vi "DriverStationPushData.vi"   [LabVIEW 2020]
doc: "This VI continously sends data from the robot to the FRC 4265 Dashboard, the joysticks, and the FIRST Driver Station. Data are only sent to the network tables when values change. Detailed sensor data are only sent when the user is currently viewing the Tune tab on the FRC 4265 Dashboard."
uses:
  04c53935-f0da-44ec-a78a-2e7adf0baac3.vi
  8f6ab1f9-5983-4917-be41-7b146f8af2a0.vi
  d6d4123b-2723-46fe-ae0c-2abe92ccdc7f.vi
  7889d354-fa55-478c-b42d-730a5990e710.vi
  09f305fd-a7e8-43a8-8a10-94883e021016.vi
  f11304fe-b25d-4509-a679-e814399fdb49.vi
  d69f5ca2-9cc8-4f10-9e43-09bf58b41655.vi
  6b66ba5c-d951-4da3-8604-42f5494a1fc8.vi
  fa6aa2a5-b57b-4d46-802a-52895c79f189.vi
  1761f515-972c-49cd-8d46-35dcec4c579e.vi
  14433321-cc0b-4c86-996a-891af0111116.vi
  665401e1-7162-4411-af45-b6d951c7e0b0.vi
  7b6a1411-5027-49fa-871d-ec9f81e31f95.vi
  20dd8ad3-6bbc-4cac-b559-7f798e2b6680.vi
  5e95d400-1295-40c5-af46-ec5444c3a2ff.vi
  d5b53c9f-0752-48c4-83e9-94c6e20357af.vi
  a2a431f6-075f-4920-bddd-4a0a2690fbc3.vi
  755407eb-a184-43a3-8213-370691478bd6.vi
  293bca24-914b-4f92-b125-1f9f12182447.vi
  63edfc8b-2713-4fb9-bbf0-712b13f7ed91.vi
  5dc304d7-e71b-4cd2-8d9d-954937278b50.vi
  c0b3d222-824d-4eea-b194-4551ccfede72.vi
  586985d1-6105-46df-bd9b-6f07d21ed352.vi
  9d68b025-fd20-40c1-968a-0b15d20a54dd.vi
  e4b3569e-220c-43b1-9843-603dbcb8d192.vi
  195aadaf-e727-4ba4-8a8c-fe9315911b93.vi
  281bad53-2b02-4799-afd8-5b44cc752506.vi
  47b7797c-6abd-448a-a8c1-ba6fc8ec09e7.vi
  fd66a432-e6c7-4ce8-9440-e2a32478c4e6.vi
  a01e8785-2e45-445a-ba95-97aad2eef7fd.vi
  b3bef00f-b543-46f7-8f0b-808f3ab90a93.vi
  6883bb39-9618-44d1-87fc-0a8820399f5c.vi
  c8eef334-f098-4cd9-9ea5-5d5092550f38.vi
  89115614-314f-44eb-b4c5-fafba5d31cd4.vi
  0c9c2ce5-4f8f-4d2f-a61f-dde9fdddd21a.vi
  948ebb5e-1fee-45f5-b788-843df8d92f11.vi
  07cec073-88f4-4f05-94a3-d05e12405c4e.vi
  c10cd8a7-bdb7-4c92-ac5c-00af4ab7dc85.vi
  f8967374-96a0-4ff7-9b39-d84b703c09a6.vi
  9891ab74-825c-4c9c-906a-dec817037994.vi
  6245c486-c412-4e37-a41a-fc8346b5d865.vi
  7dbbd9ae-9e42-48a3-962d-7503ed9ff88f.vi
  26471c2c-aca7-4047-a7cd-e40da11d04c1.vi
  15bc976b-cae7-4018-a285-3ceb7c36b13a.vi
  65b8bab8-f184-4713-b917-96f68816fcd7.vi
  e783cd06-363b-4b9f-976c-53354950d7da.vi
  423974b0-4a7b-493f-bebd-78b7d8b4919e.vi
  cbbdf295-aa1d-4db8-8566-cac5820e4458.vi
  52d993e2-6fbc-4ee4-b085-b3f80a4c3067.vi
  5ccc8aa6-325d-4660-b060-52e30b1d582a.vi
  296afef1-bc02-48ee-92b6-09523bb21575.vi
  68f74b03-6e04-47e5-994a-d14a491b94e1.vi
  811948b9-57e2-4f47-a6f6-f2932d14082f.vi
  f31b310c-46e7-4cd5-9fe8-a6567badd324.vi
  5739ca73-a30d-4c92-9c50-72d6edc45fc4.vi
  0620df73-5841-450f-a219-dd10bb38cbc0.vi
  36759aca-d9c6-44a3-918a-9a0e895c718f.vi
  d2dc3f3f-39b5-4c17-a933-05bbedc8d5d9.vi
  47e8091e-0604-4560-b6ee-932fcc40f94c.vi
  9f98788f-6f1b-4a83-a100-7d872b9f460c.vi
  d5b4d43d-cd94-4278-ad04-5030dc28ac17.vi
  cb0926b4-f1bf-44dc-b329-07cb041a7937.vi
  9304f89f-4e24-484b-bf07-7340ed265390.vi
  2e5da8e6-26da-41d5-8406-8d052fc7da1f.vi
  ea594d73-2856-44e7-ad09-a26c8a8ac1cc.vi
  bf05ee9f-e9ea-4ff1-8905-b09f1ef3a160.vi
  f39224ae-dbad-4d04-964f-bd199306b024.vi
  8b4814ac-4dea-4b6a-87df-50334cc7ef47.vi
  a59d850d-7f58-4d81-8596-951e7b208772.vi
  fb087c59-fbb1-4979-ba7d-d29f083bcd8a.vi
  040c557e-2b24-4d13-8fef-d98c711cf45f.vi
  04c53935-f0da-44ec-a78a-2e7adf0baac3.vi/77c742ae-e671-49bb-a825-a6e8cebc9f63.vi
  8f6ab1f9-5983-4917-be41-7b146f8af2a0.vi/77c742ae-e671-49bb-a825-a6e8cebc9f63.vi
  d6d4123b-2723-46fe-ae0c-2abe92ccdc7f.vi/77c742ae-e671-49bb-a825-a6e8cebc9f63.vi
  7889d354-fa55-478c-b42d-730a5990e710.vi/77c742ae-e671-49bb-a825-a6e8cebc9f63.vi
  09f305fd-a7e8-43a8-8a10-94883e021016.vi/77c742ae-e671-49bb-a825-a6e8cebc9f63.vi
  f11304fe-b25d-4509-a679-e814399fdb49.vi/77c742ae-e671-49bb-a825-a6e8cebc9f63.vi
  d69f5ca2-9cc8-4f10-9e43-09bf58b41655.vi/77c742ae-e671-49bb-a825-a6e8cebc9f63.vi
  6b66ba5c-d951-4da3-8604-42f5494a1fc8.vi/77c742ae-e671-49bb-a825-a6e8cebc9f63.vi
  fa6aa2a5-b57b-4d46-802a-52895c79f189.vi/77c742ae-e671-49bb-a825-a6e8cebc9f63.vi
  1761f515-972c-49cd-8d46-35dcec4c579e.vi/77c742ae-e671-49bb-a825-a6e8cebc9f63.vi
  14433321-cc0b-4c86-996a-891af0111116.vi/77c742ae-e671-49bb-a825-a6e8cebc9f63.vi
  665401e1-7162-4411-af45-b6d951c7e0b0.vi/77c742ae-e671-49bb-a825-a6e8cebc9f63.vi
  7b6a1411-5027-49fa-871d-ec9f81e31f95.vi/77c742ae-e671-49bb-a825-a6e8cebc9f63.vi
  20dd8ad3-6bbc-4cac-b559-7f798e2b6680.vi/77c742ae-e671-49bb-a825-a6e8cebc9f63.vi
  5e95d400-1295-40c5-af46-ec5444c3a2ff.vi/77c742ae-e671-49bb-a825-a6e8cebc9f63.vi
  d5b53c9f-0752-48c4-83e9-94c6e20357af.vi/77c742ae-e671-49bb-a825-a6e8cebc9f63.vi
  a2a431f6-075f-4920-bddd-4a0a2690fbc3.vi/77c742ae-e671-49bb-a825-a6e8cebc9f63.vi
  755407eb-a184-43a3-8213-370691478bd6.vi/77c742ae-e671-49bb-a825-a6e8cebc9f63.vi
  293bca24-914b-4f92-b125-1f9f12182447.vi/77c742ae-e671-49bb-a825-a6e8cebc9f63.vi
  63edfc8b-2713-4fb9-bbf0-712b13f7ed91.vi/77c742ae-e671-49bb-a825-a6e8cebc9f63.vi
  5dc304d7-e71b-4cd2-8d9d-954937278b50.vi/77c742ae-e671-49bb-a825-a6e8cebc9f63.vi
  586985d1-6105-46df-bd9b-6f07d21ed352.vi/77c742ae-e671-49bb-a825-a6e8cebc9f63.vi
  9d68b025-fd20-40c1-968a-0b15d20a54dd.vi/77c742ae-e671-49bb-a825-a6e8cebc9f63.vi
  e4b3569e-220c-43b1-9843-603dbcb8d192.vi/77c742ae-e671-49bb-a825-a6e8cebc9f63.vi
  195aadaf-e727-4ba4-8a8c-fe9315911b93.vi/77c742ae-e671-49bb-a825-a6e8cebc9f63.vi
  281bad53-2b02-4799-afd8-5b44cc752506.vi/77c742ae-e671-49bb-a825-a6e8cebc9f63.vi
  47b7797c-6abd-448a-a8c1-ba6fc8ec09e7.vi/77c742ae-e671-49bb-a825-a6e8cebc9f63.vi
  fd66a432-e6c7-4ce8-9440-e2a32478c4e6.vi/77c742ae-e671-49bb-a825-a6e8cebc9f63.vi
  a01e8785-2e45-445a-ba95-97aad2eef7fd.vi/77c742ae-e671-49bb-a825-a6e8cebc9f63.vi
  b3bef00f-b543-46f7-8f0b-808f3ab90a93.vi/77c742ae-e671-49bb-a825-a6e8cebc9f63.vi
  6883bb39-9618-44d1-87fc-0a8820399f5c.vi/77c742ae-e671-49bb-a825-a6e8cebc9f63.vi
  c8eef334-f098-4cd9-9ea5-5d5092550f38.vi/77c742ae-e671-49bb-a825-a6e8cebc9f63.vi
  89115614-314f-44eb-b4c5-fafba5d31cd4.vi/77c742ae-e671-49bb-a825-a6e8cebc9f63.vi
  0c9c2ce5-4f8f-4d2f-a61f-dde9fdddd21a.vi/77c742ae-e671-49bb-a825-a6e8cebc9f63.vi
  948ebb5e-1fee-45f5-b788-843df8d92f11.vi/77c742ae-e671-49bb-a825-a6e8cebc9f63.vi
  07cec073-88f4-4f05-94a3-d05e12405c4e.vi/77c742ae-e671-49bb-a825-a6e8cebc9f63.vi
  c10cd8a7-bdb7-4c92-ac5c-00af4ab7dc85.vi/77c742ae-e671-49bb-a825-a6e8cebc9f63.vi
  f8967374-96a0-4ff7-9b39-d84b703c09a6.vi/77c742ae-e671-49bb-a825-a6e8cebc9f63.vi
  9891ab74-825c-4c9c-906a-dec817037994.vi/77c742ae-e671-49bb-a825-a6e8cebc9f63.vi
  6245c486-c412-4e37-a41a-fc8346b5d865.vi/77c742ae-e671-49bb-a825-a6e8cebc9f63.vi
  7dbbd9ae-9e42-48a3-962d-7503ed9ff88f.vi/77c742ae-e671-49bb-a825-a6e8cebc9f63.vi
  26471c2c-aca7-4047-a7cd-e40da11d04c1.vi/77c742ae-e671-49bb-a825-a6e8cebc9f63.vi
  15bc976b-cae7-4018-a285-3ceb7c36b13a.vi/77c742ae-e671-49bb-a825-a6e8cebc9f63.vi
  65b8bab8-f184-4713-b917-96f68816fcd7.vi/77c742ae-e671-49bb-a825-a6e8cebc9f63.vi
  e783cd06-363b-4b9f-976c-53354950d7da.vi/77c742ae-e671-49bb-a825-a6e8cebc9f63.vi
  423974b0-4a7b-493f-bebd-78b7d8b4919e.vi/77c742ae-e671-49bb-a825-a6e8cebc9f63.vi
  cbbdf295-aa1d-4db8-8566-cac5820e4458.vi/77c742ae-e671-49bb-a825-a6e8cebc9f63.vi
  52d993e2-6fbc-4ee4-b085-b3f80a4c3067.vi/77c742ae-e671-49bb-a825-a6e8cebc9f63.vi
  5ccc8aa6-325d-4660-b060-52e30b1d582a.vi/77c742ae-e671-49bb-a825-a6e8cebc9f63.vi
  296afef1-bc02-48ee-92b6-09523bb21575.vi/77c742ae-e671-49bb-a825-a6e8cebc9f63.vi
  68f74b03-6e04-47e5-994a-d14a491b94e1.vi/77c742ae-e671-49bb-a825-a6e8cebc9f63.vi
  811948b9-57e2-4f47-a6f6-f2932d14082f.vi/77c742ae-e671-49bb-a825-a6e8cebc9f63.vi
  f31b310c-46e7-4cd5-9fe8-a6567badd324.vi/77c742ae-e671-49bb-a825-a6e8cebc9f63.vi
  5739ca73-a30d-4c92-9c50-72d6edc45fc4.vi/77c742ae-e671-49bb-a825-a6e8cebc9f63.vi
  0620df73-5841-450f-a219-dd10bb38cbc0.vi/77c742ae-e671-49bb-a825-a6e8cebc9f63.vi
  36759aca-d9c6-44a3-918a-9a0e895c718f.vi/77c742ae-e671-49bb-a825-a6e8cebc9f63.vi
  d2dc3f3f-39b5-4c17-a933-05bbedc8d5d9.vi/77c742ae-e671-49bb-a825-a6e8cebc9f63.vi
  47e8091e-0604-4560-b6ee-932fcc40f94c.vi/77c742ae-e671-49bb-a825-a6e8cebc9f63.vi
  9f98788f-6f1b-4a83-a100-7d872b9f460c.vi/77c742ae-e671-49bb-a825-a6e8cebc9f63.vi
  d5b4d43d-cd94-4278-ad04-5030dc28ac17.vi/77c742ae-e671-49bb-a825-a6e8cebc9f63.vi
  cb0926b4-f1bf-44dc-b329-07cb041a7937.vi/77c742ae-e671-49bb-a825-a6e8cebc9f63.vi
  9304f89f-4e24-484b-bf07-7340ed265390.vi/77c742ae-e671-49bb-a825-a6e8cebc9f63.vi
  2e5da8e6-26da-41d5-8406-8d052fc7da1f.vi/77c742ae-e671-49bb-a825-a6e8cebc9f63.vi
  ea594d73-2856-44e7-ad09-a26c8a8ac1cc.vi/77c742ae-e671-49bb-a825-a6e8cebc9f63.vi
  bf05ee9f-e9ea-4ff1-8905-b09f1ef3a160.vi/77c742ae-e671-49bb-a825-a6e8cebc9f63.vi
  f39224ae-dbad-4d04-964f-bd199306b024.vi/77c742ae-e671-49bb-a825-a6e8cebc9f63.vi
  8b4814ac-4dea-4b6a-87df-50334cc7ef47.vi/77c742ae-e671-49bb-a825-a6e8cebc9f63.vi
  a59d850d-7f58-4d81-8596-951e7b208772.vi/77c742ae-e671-49bb-a825-a6e8cebc9f63.vi
  fb087c59-fbb1-4979-ba7d-d29f083bcd8a.vi/77c742ae-e671-49bb-a825-a6e8cebc9f63.vi
  040c557e-2b24-4d13-8fef-d98c711cf45f.vi/77c742ae-e671-49bb-a825-a6e8cebc9f63.vi
  driverdata.vi
  <vilib>/Rock Robotics/Network Tables/NT Write String.vi
  sensordata.vi
  <vilib>/Rock Robotics/Network Tables/NT Write Boolean.vi
  robotconstants.vi
  <vilib>/Rock Robotics/Network Tables/NT Write String Array.vi
  autonomousinfo.vi
  <vilib>/Rock Robotics/Network Tables/NT Write Number.vi
  robotoutputs.vi
  <vilib>/Rock Robotics/Network Tables/NT Write Numeric Array.vi
  <vilib>/Rock Robotics/Network Tables/NT Write Boolean Array.vi
  robotprofiles.vi
types:
  T1 = typedef "WPI_DriverStationAllianceInfo.ctl" = enum16{"Red", "Blue", "Invalid"}
  T2 = typedef "WPI_DriverStationRobotMode2.ctl" = enum16{"Autonomous Disabled", "Autonomous Enabled", "Teleop Disabled", "Teleop Enabled", "Disconnected", "Finish", "Test Disabled", "Test Enabled", "Emergency Stopped"}
  T3 = enum16{"Low Gear", "High Gear", "Transiting", "Unknown", "Force Low Gear"}
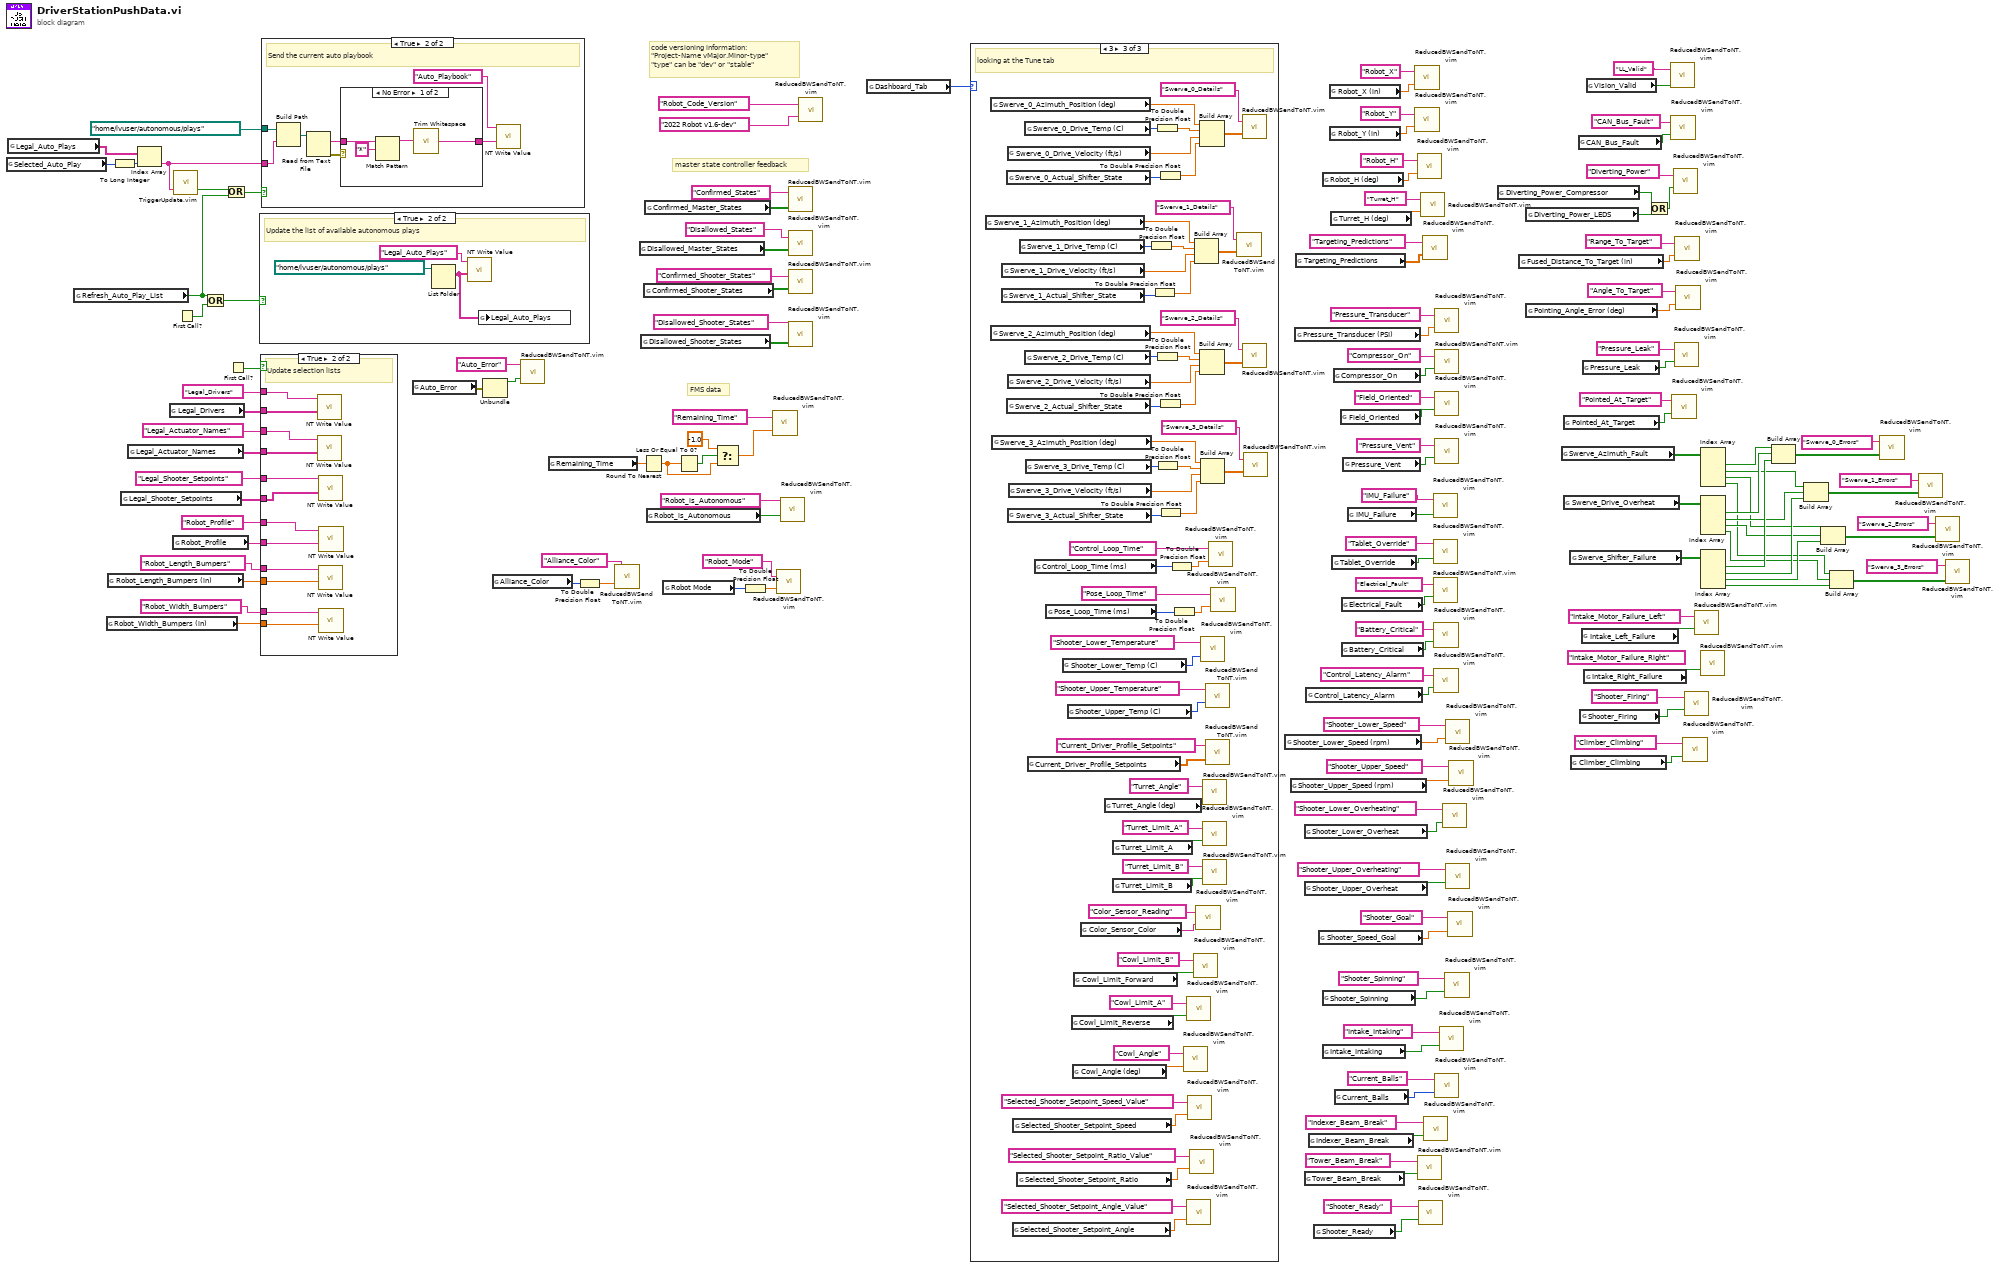
[diagram p0: block diagram]
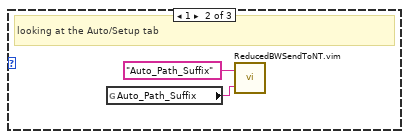
[diagram p3: hidden frame]
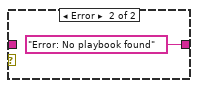
[diagram p6: hidden frame]
diagram:
  (unwired) "Intake_Motor_Failure_Right" ("Name")
  # "FMS data"
  # "master state controller feedback"
  # "code versioning information:\n\"Project-Name vMajor.Minor-type\"\n\"type\" can be \"dev\" or \"stable\""
  n1 = global read "driverdata.vi" "Selected_Auto_Play"() -> (w141:u16)
  n2 = global read "robotconstants.vi" "Legal_Auto_Plays"() -> (w136:string[])
  n3 = global read "driverdata.vi" "Refresh_Auto_Play_List"() -> (w137:bool)
  n4 = global read "robotconstants.vi" "Robot_Width_Bumpers (in)"() -> (w3:dbl)
  n5 = global read "robotconstants.vi" "Robot_Length_Bumpers (in)"() -> (w6:dbl)
  n6 = To Long Integer(number=w141) -> (32bit integer=w142:i32)
  n7 = global read "robotconstants.vi" "Legal_Shooter_Setpoints"() -> (w129:string[])
  n8 = global read "robotconstants.vi" "Legal_Actuator_Names"() -> (w130:string[])
  n9 = Index Array(array=w136, index=w142) -> (element=w140:string)
  n10 = global read "robotconstants.vi" "Legal_Drivers"() -> (w23:string[])
  n11 = global read "robotprofiles.vi" "Robot_Profile"() -> (w22:string)
  n12 = call "TriggerUpdate.vim"("Trigger"=w140) -> ("Update"=w139:bool)  [unwired: 2 in]
  n13 = First Call?() -> (First Call?: T/F=w145:bool)
  n14 = Or(x=w137, y=w145) -> (x .or. y?=w144:bool)
  n15 = Or(x=w139, y=w137) -> (x .or. y?=w138:bool)
  n16 = First Call?() -> (First Call?: T/F=w134:bool)
  n17 = case shown="True" w144 {
    frame False {
    }
    frame True {
      # "Update the list of available autonomous plays"
      n18 = List Folder(path=path "/home/lvuser/autonomous/plays") -> (filenames=w148:string[])  [unwired: 3 in, 3 out]
      n19 = call-poly <vilib>:"NT Write Value.vi"("String Array"=w148, "Name"="Legal_Auto_Plays") -> ()  [unwired: 9 in, 1 out]
      n20 = global write "robotconstants.vi" "Legal_Auto_Plays"(w148) -> ()
    }
  }
  n21 = case shown="True" w134 {
    tunnel: "Legal_Drivers" ("Name") -> [_ w162]
    tunnel: w130 -> [_ w161]
    tunnel: "Legal_Actuator_Names" ("Name") -> [_ w160]
    tunnel: "Robot_Profile" ("Name") -> [_ w159]
    tunnel: w22 -> [_ w158]
    tunnel: "Legal_Shooter_Setpoints" ("Name") -> [_ w157]
    tunnel: w129 -> [_ w156]
    tunnel: w23 -> [_ w155]
    tunnel: w6 -> [_ w154]
    tunnel: "Robot_Length_Bumpers" ("Name") -> [_ w153]
    tunnel: "Robot_Width_Bumpers" ("Name") -> [_ w152]
    tunnel: w3 -> [_ w151]
    frame False {
    }
    frame True {
      # "Update selection lists"
      n22 = call-poly <vilib>:"NT Write Value.vi"("String Array"=w155, "Name"=w162) -> ()  [unwired: 9 in, 1 out]
      n23 = call-poly <vilib>:"NT Write Value.vi"("String Array"=w161, "Name"=w160) -> ()  [unwired: 9 in, 1 out]
      n24 = call-poly <vilib>:"NT Write Value.vi"("String Array"=w156, "Name"=w157) -> ()  [unwired: 9 in, 1 out]
      n25 = call-poly <vilib>:"NT Write Value.vi"("Numeric"=w154, "Name"=w153) -> ()  [unwired: 9 in, 1 out]
      n26 = call-poly <vilib>:"NT Write Value.vi"("String"=w158, "Name"=w159) -> ()  [unwired: 9 in, 1 out]
      n27 = call-poly <vilib>:"NT Write Value.vi"("Numeric"=w151, "Name"=w152) -> ()  [unwired: 9 in, 1 out]
    }
  }
  n28 = case shown="True" w138 {
    tunnel: path "/home/lvuser/autonomous/plays" ("path") -> [_ w169]
    tunnel: w140 -> [_ w165]
    frame False {
    }
    frame True {
      # "Send the current auto playbook"
      n29 = Build Path(base path=w169, name or relative path=w165) -> (appended path=w168:path)
      n30 = Read from Text File(file (use dialog)=w168) -> (text=w166:string, error out=w167:errorcluster)  [unwired: 3 in, 2 out]
      n31 = case shown="No Error" w167 {
        tunnel: w166 -> [w173 _]
        tunnel: [w172 "Error: No playbook found"] -> w164
        frame No Error {
          n32 = Match Pattern(string=w173, regular expression="*") -> (before substring=w170:string)  [unwired: 1 in, 3 out]
          n33 = call <vilib>:"Trim Whitespace.vi"("string"=w170) -> ("trimmed string"=w172:string)  [unwired: 1 in]
        }
        frame Error {
        }
      }
      n34 = call-poly <vilib>:"NT Write Value.vi"("String"=w164, "Name"="Auto_Playbook") -> ()  [unwired: 9 in, 1 out]
    }
  }
  n35 = global read "autonomousinfo.vi" "Auto_Error"() -> (w128:errorcluster)
  n36 = Unbundle(w128) -> ("status"=w126:bool)  [unwired: 2 out]
  n37 = global read "driverdata.vi" "Alliance_Color"() -> (w28:T1)
  n38 = call "ReducedBWSendToNT.vim"("Value In"=w126, "NT Name"="Auto_Error" ("Name")) -> ()  [unwired: 1 out]
  n39 = global read "driverdata.vi" "Remaining_Time"() -> (w27:dbl)
  n40 = To Double Precision Float(number=w28) -> (double precision float=w30:dbl)
  n41 = call "ReducedBWSendToNT.vim"("Value In"=w30, "NT Name"="Alliance_Color") -> ()  [unwired: 1 out]
  n42 = global read "robotoutputs.vi" "Disallowed_Master_States"() -> (w42:bool[])
  n43 = global read "robotoutputs.vi" "Disallowed_Shooter_States"() -> (w38:bool[])
  n44 = Round To Nearest(number=w27) -> (nearest integer value=w120:dbl)
  n45 = global read "robotoutputs.vi" "Confirmed_Shooter_States"() -> (w40:bool[])
  n46 = global read "robotoutputs.vi" "Confirmed_Master_States"() -> (w44:bool[])
  n47 = global read "driverdata.vi" "Robot_is_Autonomous"() -> (w118:bool)
  n48 = global read "driverdata.vi" "Robot Mode"() -> (w26:T2)
  n49 = Less Or Equal To 0?(x=w120) -> (x <= 0?=w123:bool)
  n50 = Select(t=-1.0, s=w123, f=w120) -> (s? t:f=w24:dbl)
  n51 = To Double Precision Float(number=w26) -> (double precision float=w25:dbl)
  n52 = call "ReducedBWSendToNT.vim"("Value In"=w24, "NT Name"="Remaining_Time" ("Name")) -> ()  [unwired: 1 out]
  n53 = call "ReducedBWSendToNT.vim"("Value In"=w25, "NT Name"="Robot_Mode") -> ()  [unwired: 1 out]
  n54 = call "ReducedBWSendToNT.vim"("Value In"=w118, "NT Name"="Robot_is_Autonomous") -> ()  [unwired: 1 out]
  n55 = call "ReducedBWSendToNT.vim"("Value In"=w44, "NT Name"="Confirmed_States" ("Name")) -> ()  [unwired: 1 out]
  n56 = call "ReducedBWSendToNT.vim"("Value In"=w42, "NT Name"="Disallowed_States" ("Name")) -> ()  [unwired: 1 out]
  n57 = call "ReducedBWSendToNT.vim"("Value In"=w40, "NT Name"="Confirmed_Shooter_States" ("Name")) -> ()  [unwired: 1 out]
  n58 = call "ReducedBWSendToNT.vim"("Value In"=w38, "NT Name"="Disallowed_Shooter_States" ("Name")) -> ()  [unwired: 1 out]
  n59 = call "ReducedBWSendToNT.vim"("Value In"="2022 Robot v1.6-dev", "NT Name"="Robot_Code_Version" ("Name")) -> ()  [unwired: 1 out]
  n60 = global read "driverdata.vi" "Dashboard_Tab"() -> (w37:i8)
  n61 = case shown="3" w37 {
    frame 0, Default {
      # "not looking at a specific tab"
    }
    frame 1 {
      # "looking at the Auto/Setup tab"
      n62 = global read "autonomousinfo.vi" "Auto_Path_Suffix"() -> (w176:string)
      n63 = call "ReducedBWSendToNT.vim"("Value In"=w176, "NT Name"="Auto_Path_Suffix" ("Name")) -> ()  [unwired: 1 out]
    }
    frame 3 {
      # "looking at the Tune tab"
      n64 = global read "sensordata.vi" "Swerve_1_Azimuth_Position (deg)"() -> (w220:dbl)
      n65 = global read "sensordata.vi" "Swerve_0_Azimuth_Position (deg)"() -> (w228:dbl)
      n66 = global read "sensordata.vi" "Swerve_2_Azimuth_Position (deg)"() -> (w212:dbl)
      n67 = global read "sensordata.vi" "Swerve_3_Azimuth_Position (deg)"() -> (w204:dbl)
      n68 = global read "sensordata.vi" "Swerve_1_Actual_Shifter_State"() -> (w216:T3)
      n69 = global read "sensordata.vi" "Swerve_1_Drive_Velocity (ft/s)"() -> (w219:dbl)
      n70 = global read "sensordata.vi" "Swerve_0_Actual_Shifter_State"() -> (w224:T3)
      n71 = global read "sensordata.vi" "Swerve_2_Actual_Shifter_State"() -> (w208:T3)
      n72 = global read "sensordata.vi" "Swerve_0_Drive_Velocity (ft/s)"() -> (w227:dbl)
      n73 = global read "sensordata.vi" "Swerve_2_Drive_Velocity (ft/s)"() -> (w211:dbl)
      n74 = global read "sensordata.vi" "Swerve_3_Actual_Shifter_State"() -> (w200:T3)
      n75 = global read "sensordata.vi" "Swerve_3_Drive_Velocity (ft/s)"() -> (w203:dbl)
      n76 = global read "robotoutputs.vi" "Selected_Shooter_Setpoint_Angle"() -> (w177:dbl)
      n77 = global read "robotoutputs.vi" "Selected_Shooter_Setpoint_Speed"() -> (w181:dbl)
      n78 = global read "robotoutputs.vi" "Selected_Shooter_Setpoint_Ratio"() -> (w179:dbl)
      n79 = global read "sensordata.vi" "Swerve_1_Drive_Temp (C)"() -> (w218:u8)
      n80 = global read "sensordata.vi" "Swerve_0_Drive_Temp (C)"() -> (w226:u8)
      n81 = global read "sensordata.vi" "Swerve_2_Drive_Temp (C)"() -> (w210:u8)
      n82 = global read "sensordata.vi" "Swerve_3_Drive_Temp (C)"() -> (w202:u8)
      n83 = global read "robotoutputs.vi" "Current_Driver_Profile_Setpoints"() -> (w230:dbl[])
      n84 = global read "sensordata.vi" "Control_Loop_Time (ms)"() -> (w240:u32)
      n85 = global read "sensordata.vi" "Pose_Loop_Time (ms)"() -> (w237:u32)
      n86 = global read "sensordata.vi" "Shooter_Lower_Temp (C)"() -> (w234:u8)
      n87 = global read "sensordata.vi" "Shooter_Upper_Temp (C)"() -> (w232:u8)
      n88 = global read "sensordata.vi" "Cowl_Limit_Reverse"() -> (w185:bool)
      n89 = global read "sensordata.vi" "Cowl_Angle (deg)"() -> (w184:dbl)
      n90 = global read "sensordata.vi" "Cowl_Limit_Forward"() -> (w187:bool)
      n91 = global read "sensordata.vi" "Color_Sensor_Color"() -> (w190:string)
      n92 = global read "sensordata.vi" "Turret_Angle (deg)"() -> (w196:dbl)
      n93 = global read "sensordata.vi" "Turret_Limit_A"() -> (w194:bool)
      n94 = global read "sensordata.vi" "Turret_Limit_B"() -> (w192:bool)
      n95 = To Double Precision Float(number=w218) -> (double precision float=w217:dbl)
      n96 = To Double Precision Float(number=w216) -> (double precision float=w215:dbl)
      n97 = To Double Precision Float(number=w226) -> (double precision float=w225:dbl)
      n98 = To Double Precision Float(number=w210) -> (double precision float=w209:dbl)
      n99 = To Double Precision Float(number=w202) -> (double precision float=w201:dbl)
      n100 = To Double Precision Float(number=w224) -> (double precision float=w223:dbl)
      n101 = To Double Precision Float(number=w208) -> (double precision float=w207:dbl)
      n102 = To Double Precision Float(number=w200) -> (double precision float=w199:dbl)
      n103 = To Double Precision Float(number=w240) -> (double precision float=w238:dbl)
      n104 = To Double Precision Float(number=w237) -> (double precision float=w235:dbl)
      n105 = call "ReducedBWSendToNT.vim"("Value In"=w184, "NT Name"="Cowl_Angle" ("Name")) -> ()  [unwired: 1 out]
      n106 = call "ReducedBWSendToNT.vim"("Value In"=w185, "NT Name"="Cowl_Limit_A" ("Name")) -> ()  [unwired: 1 out]
      n107 = call "ReducedBWSendToNT.vim"("Value In"=w177, "NT Name"="Selected_Shooter_Setpoint_Angle_Value" ("Name")) -> ()  [unwired: 1 out]
      n108 = call "ReducedBWSendToNT.vim"("Value In"=w181, "NT Name"="Selected_Shooter_Setpoint_Speed_Value" ("Name")) -> ()  [unwired: 1 out]
      n109 = call "ReducedBWSendToNT.vim"("Value In"=w179, "NT Name"="Selected_Shooter_Setpoint_Ratio_Value" ("Name")) -> ()  [unwired: 1 out]
      n110 = call "ReducedBWSendToNT.vim"("Value In"=w187, "NT Name"="Cowl_Limit_B" ("Name")) -> ()  [unwired: 1 out]
      n111 = Build Array(w220, w217, w219, w215) -> (w214:dbl[])
      n112 = call "ReducedBWSendToNT.vim"("Value In"=w190, "NT Name"="Color_Sensor_Reading" ("Name")) -> ()  [unwired: 1 out]
      n113 = Build Array(w228, w225, w227, w223) -> (w222:dbl[])
      n114 = Build Array(w212, w209, w211, w207) -> (w206:dbl[])
      n115 = Build Array(w204, w201, w203, w199) -> (w198:dbl[])
      n116 = call "ReducedBWSendToNT.vim"("Value In"=w234, "NT Name"="Shooter_Lower_Temperature" ("Name")) -> ()  [unwired: 1 out]
      n117 = call "ReducedBWSendToNT.vim"("Value In"=w196, "NT Name"="Turret_Angle" ("Name")) -> ()  [unwired: 1 out]
      n118 = call "ReducedBWSendToNT.vim"("Value In"=w194, "NT Name"="Turret_Limit_A" ("Name")) -> ()  [unwired: 1 out]
      n119 = call "ReducedBWSendToNT.vim"("Value In"=w192, "NT Name"="Turret_Limit_B" ("Name")) -> ()  [unwired: 1 out]
      n120 = call "ReducedBWSendToNT.vim"("Value In"=w232, "NT Name"="Shooter_Upper_Temperature" ("Name")) -> ()  [unwired: 1 out]
      n121 = call "ReducedBWSendToNT.vim"("Value In"=w230, "NT Name"="Current_Driver_Profile_Setpoints" ("Name")) -> ()  [unwired: 1 out]
      n122 = call "ReducedBWSendToNT.vim"("Value In"=w238, "NT Name"="Control_Loop_Time" ("Name")) -> ()  [unwired: 1 out]
      n123 = call "ReducedBWSendToNT.vim"("Value In"=w235, "NT Name"="Pose_Loop_Time" ("Name")) -> ()  [unwired: 1 out]
      n124 = call "ReducedBWSendToNT.vim"("Value In"=w214, "NT Name"="Swerve_1_Details") -> ()  [unwired: 1 out]
      n125 = call "ReducedBWSendToNT.vim"("Value In"=w222, "NT Name"="Swerve_0_Details") -> ()  [unwired: 1 out]
      n126 = call "ReducedBWSendToNT.vim"("Value In"=w206, "NT Name"="Swerve_2_Details") -> ()  [unwired: 1 out]
      n127 = call "ReducedBWSendToNT.vim"("Value In"=w198, "NT Name"="Swerve_3_Details") -> ()  [unwired: 1 out]
    }
  }
  n128 = global read "sensordata.vi" "Shooter_Lower_Speed (rpm)"() -> (w83:dbl)
  n129 = global read "sensordata.vi" "Shooter_Upper_Speed (rpm)"() -> (w81:dbl)
  n130 = global read "sensordata.vi" "Pressure_Transducer (PSI)"() -> (w111:dbl)
  n131 = global read "sensordata.vi" "Targeting_Predictions"() -> (w35:dbl[])
  n132 = global read "sensordata.vi" "Shooter_Lower_Overheat"() -> (w80:bool)
  n133 = global read "sensordata.vi" "Shooter_Upper_Overheat"() -> (w74:bool)
  n134 = global read "sensordata.vi" "Tower_Beam_Break"() -> (w15:bool)
  n135 = global read "sensordata.vi" "Control_Latency_Alarm"() -> (w92:bool)
  n136 = global read "sensordata.vi" "Indexer_Beam_Break"() -> (w17:bool)
  n137 = global read "robotoutputs.vi" "Shooter_Ready"() -> (w12:bool)
  n138 = global read "robotoutputs.vi" "Shooter_Speed_Goal"() -> (w71:dbl)
  n139 = global read "sensordata.vi" "Robot_H (deg)"() -> (w34:dbl)
  n140 = global read "robotoutputs.vi" "Shooter_Spinning"() -> (w69:bool)
  n141 = global read "robotoutputs.vi" "Intake_Intaking"() -> (w20:bool)
  n142 = global read "sensordata.vi" "Robot_X (in)"() -> (w115:dbl)
  n143 = global read "sensordata.vi" "Robot_Y (in)"() -> (w113:dbl)
  n144 = global read "sensordata.vi" "Turret_H (deg)"() -> (w36:dbl)
  n145 = global read "driverdata.vi" "Tablet_Override"() -> (w98:bool)
  n146 = global read "sensordata.vi" "Compressor_On"() -> (w109:bool)
  n147 = global read "sensordata.vi" "Current_Balls"() -> (w18:i32)
  n148 = global read "robotoutputs.vi" "Field_Oriented"() -> (w107:bool)
  n149 = global read "sensordata.vi" "Electrical_Fault"() -> (w96:bool)
  n150 = global read "sensordata.vi" "Battery_Critical"() -> (w94:bool)
  n151 = global read "sensordata.vi" "Pressure_Vent"() -> (w105:bool)
  n152 = global read "sensordata.vi" "IMU_Failure"() -> (w100:bool)
  n153 = call "ReducedBWSendToNT.vim"("Value In"=w115, "NT Name"="Robot_X" ("Name")) -> ()  [unwired: 1 out]
  n154 = call "ReducedBWSendToNT.vim"("Value In"=w113, "NT Name"="Robot_Y" ("Name")) -> ()  [unwired: 1 out]
  n155 = call "ReducedBWSendToNT.vim"("Value In"=w34, "NT Name"="Robot_H" ("Name")) -> ()  [unwired: 1 out]
  n156 = call "ReducedBWSendToNT.vim"("Value In"=w15, "NT Name"="Tower_Beam_Break" ("Name")) -> ()  [unwired: 1 out]
  n157 = call "ReducedBWSendToNT.vim"("Value In"=w12, "NT Name"="Shooter_Ready" ("Name")) -> ()  [unwired: 1 out]
  n158 = call "ReducedBWSendToNT.vim"("Value In"=w36, "NT Name"="Turret_H" ("Name")) -> ()  [unwired: 1 out]
  n159 = call "ReducedBWSendToNT.vim"("Value In"=w35, "NT Name"="Targeting_Predictions" ("Name")) -> ()  [unwired: 1 out]
  n160 = call "ReducedBWSendToNT.vim"("Value In"=w17, "NT Name"="Indexer_Beam_Break" ("Name")) -> ()  [unwired: 1 out]
  n161 = call "ReducedBWSendToNT.vim"("Value In"=w100, "NT Name"="IMU_Failure" ("Name")) -> ()  [unwired: 1 out]
  n162 = call "ReducedBWSendToNT.vim"("Value In"=w98, "NT Name"="Tablet_Override" ("Name")) -> ()  [unwired: 1 out]
  n163 = call "ReducedBWSendToNT.vim"("Value In"=w96, "NT Name"="Electrical_Fault" ("Name")) -> ()  [unwired: 1 out]
  n164 = call "ReducedBWSendToNT.vim"("Value In"=w94, "NT Name"="Battery_Critical" ("Name")) -> ()  [unwired: 1 out]
  n165 = call "ReducedBWSendToNT.vim"("Value In"=w92, "NT Name"="Control_Latency_Alarm" ("Name")) -> ()  [unwired: 1 out]
  n166 = call "ReducedBWSendToNT.vim"("Value In"=w111, "NT Name"="Pressure_Transducer" ("Name")) -> ()  [unwired: 1 out]
  n167 = call "ReducedBWSendToNT.vim"("Value In"=w109, "NT Name"="Compressor_On" ("Name")) -> ()  [unwired: 1 out]
  n168 = call "ReducedBWSendToNT.vim"("Value In"=w107, "NT Name"="Field_Oriented" ("Name")) -> ()  [unwired: 1 out]
  n169 = call "ReducedBWSendToNT.vim"("Value In"=w105, "NT Name"="Pressure_Vent" ("Name")) -> ()  [unwired: 1 out]
  n170 = call "ReducedBWSendToNT.vim"("Value In"=w18, "NT Name"="Current_Balls" ("Name")) -> ()  [unwired: 1 out]
  n171 = call "ReducedBWSendToNT.vim"("Value In"=w20, "NT Name"="Intake_Intaking" ("Name")) -> ()  [unwired: 1 out]
  n172 = call "ReducedBWSendToNT.vim"("Value In"=w80, "NT Name"="Shooter_Lower_Overheating" ("Name")) -> ()  [unwired: 1 out]
  n173 = call "ReducedBWSendToNT.vim"("Value In"=w69, "NT Name"="Shooter_Spinning" ("Name")) -> ()  [unwired: 1 out]
  n174 = call "ReducedBWSendToNT.vim"("Value In"=w83, "NT Name"="Shooter_Lower_Speed" ("Name")) -> ()  [unwired: 1 out]
  n175 = call "ReducedBWSendToNT.vim"("Value In"=w74, "NT Name"="Shooter_Upper_Overheating" ("Name")) -> ()  [unwired: 1 out]
  n176 = call "ReducedBWSendToNT.vim"("Value In"=w71, "NT Name"="Shooter_Goal" ("Name")) -> ()  [unwired: 1 out]
  n177 = call "ReducedBWSendToNT.vim"("Value In"=w81, "NT Name"="Shooter_Upper_Speed" ("Name")) -> ()  [unwired: 1 out]
  n178 = global read "robotoutputs.vi" "Diverting_Power_Compressor"() -> (w90:bool)
  n179 = global read "sensordata.vi" "Fused_Distance_To_Target (in)"() -> (w102:dbl)
  n180 = global read "robotoutputs.vi" "Diverting_Power_LEDS"() -> (w89:bool)
  n181 = global read "sensordata.vi" "Pointing_Angle_Error (deg)"() -> (w75:dbl)
  n182 = global read "sensordata.vi" "Swerve_Azimuth_Fault"() -> (w68:bool[])
  n183 = global read "sensordata.vi" "Pointed_At_Target"() -> (w85:bool)
  n184 = global read "sensordata.vi" "Swerve_Drive_Overheat"() -> (w67:bool[])
  n185 = global read "sensordata.vi" "Swerve_Shifter_Failure"() -> (w66:bool[])
  n186 = global read "robotoutputs.vi" "Climber_Climbing"() -> (w1:bool)
  n187 = global read "sensordata.vi" "CAN_Bus_Fault"() -> (w87:bool)
  n188 = global read "robotoutputs.vi" "Shooter_Firing"() -> (w7:bool)
  n189 = global read "sensordata.vi" "Intake_Left_Failure"() -> (w10:bool)
  n190 = global read "sensordata.vi" "Pressure_Leak"() -> (w77:bool)
  n191 = global read "sensordata.vi" "Intake_Right_Failure"() -> (w9:bool)
  n192 = global read "sensordata.vi" "Vision_Valid"() -> (w146:bool)
  n193 = Or(x=w90, y=w89) -> (x .or. y?=w91:bool)
  n194 = call "ReducedBWSendToNT.vim"("Value In"=w146, "NT Name"="LL_Valid" ("Name")) -> ()  [unwired: 1 out]
  n195 = call "ReducedBWSendToNT.vim"("Value In"=w87, "NT Name"="CAN_Bus_Fault" ("Name")) -> ()  [unwired: 1 out]
  n196 = call "ReducedBWSendToNT.vim"("Value In"=w85, "NT Name"="Pointed_At_Target" ("Name")) -> ()  [unwired: 1 out]
  n197 = call "ReducedBWSendToNT.vim"("Value In"=w91, "NT Name"="Diverting_Power" ("Name")) -> ()  [unwired: 1 out]
  n198 = call "ReducedBWSendToNT.vim"("Value In"=w77, "NT Name"="Pressure_Leak" ("Name")) -> ()  [unwired: 1 out]
  n199 = call "ReducedBWSendToNT.vim"("Value In"=w102, "NT Name"="Range_To_Target" ("Name")) -> ()  [unwired: 1 out]
  n200 = call "ReducedBWSendToNT.vim"("Value In"=w75, "NT Name"="Angle_To_Target" ("Name")) -> ()  [unwired: 1 out]
  n201 = call "ReducedBWSendToNT.vim"("Value In"=w1, "NT Name"="Climber_Climbing" ("Name")) -> ()  [unwired: 1 out]
  n202 = call "ReducedBWSendToNT.vim"("Value In"=w7, "NT Name"="Shooter_Firing" ("Name")) -> ()  [unwired: 1 out]
  n203 = call "ReducedBWSendToNT.vim"("Value In"=w10, "NT Name"="Intake_Motor_Failure_Left" ("Name")) -> ()  [unwired: 1 out]
  n204 = call "ReducedBWSendToNT.vim"("Value In"=w9) -> ()  [unwired: 1 in, 1 out]
  n205 = Index Array(array=w68) -> (element #1=w65:bool, element #2=w62:bool, element #3=w59:bool, element #4=w56:bool)  [unwired: 4 in]
  n206 = Index Array(array=w67) -> (element #1=w64:bool, element #2=w61:bool, element #3=w58:bool, element #4=w55:bool)  [unwired: 4 in]
  n207 = Index Array(array=w66) -> (element #1=w63:bool, element #2=w60:bool, element #3=w57:bool, element #4=w54:bool)  [unwired: 4 in]
  n208 = Build Array(w65, w64, w63) -> (w53:bool[])
  n209 = Build Array(w62, w61, w60) -> (w50:bool[])
  n210 = Build Array(w59, w58, w57) -> (w48:bool[])
  n211 = Build Array(w56, w55, w54) -> (w46:bool[])
  n212 = call "ReducedBWSendToNT.vim"("Value In"=w53, "NT Name"="Swerve_0_Errors") -> ()  [unwired: 1 out]
  n213 = call "ReducedBWSendToNT.vim"("Value In"=w50, "NT Name"="Swerve_1_Errors") -> ()  [unwired: 1 out]
  n214 = call "ReducedBWSendToNT.vim"("Value In"=w48, "NT Name"="Swerve_2_Errors") -> ()  [unwired: 1 out]
  n215 = call "ReducedBWSendToNT.vim"("Value In"=w46, "NT Name"="Swerve_3_Errors") -> ()  [unwired: 1 out]
